vi "PythonFacadeTest.vi"(0 "Data In":T4={"VISA Refnum in"="", "All Code"="Hi"}, 2 "Display State In":T2, 3 "Container State":T3) -> (6 "Data Out":T4={"VISA Refnum in"="", "All Code"="Hi"}, 7 "Display State Out":T2, 8 "Action":T1)   [LabVIEW 2016]
uses:
  <vilib>/_xctls/Action.ctl
  <vilib>/_xctls/XControlSupport.lvlib
  uPythonX.xctl
  <vilib>/_xctls/Container State.ctl
  PythonData.ctl
  PythonState.ctl
panel:
  in  "View":u16(ring)
  in  "SubCode":string
  in  "Save on MP":bool
  in  "REPL":bool
  out "Port":string
  in  "Help":bool
  in  "Python":T5
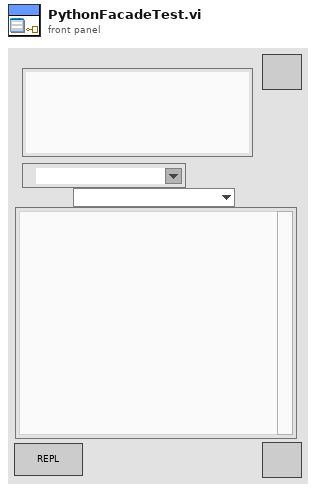
[diagram p1: front panel]
types:
  T1 = typedef "XControlSupport.lvlib/Action.ctl" = cluster{"Data Changed?":bool, "State Changed?":bool, "Action Name":string}
  T2 = typedef "uPythonX.xctl/PythonState.ctl" = cluster{"Numeric":dbl}
  T3 = typedef "XControlSupport.lvlib/Container State.ctl" = cluster{"Indicator?":bool, "Run Mode?":bool, " Refnum":refnum<vi>}
  T4 = typedef "uPythonX.xctl/PythonData.ctl" = cluster{"VISA Refnum in":refnum<visa-resource-name>, "All Code":string}
  T5 = cluster{"VISA in":refnum<visa-resource-name>, "Code":string}
  T6 = cluster{"SubCode":refnum<vi>, "Panel":refnum<vi>}
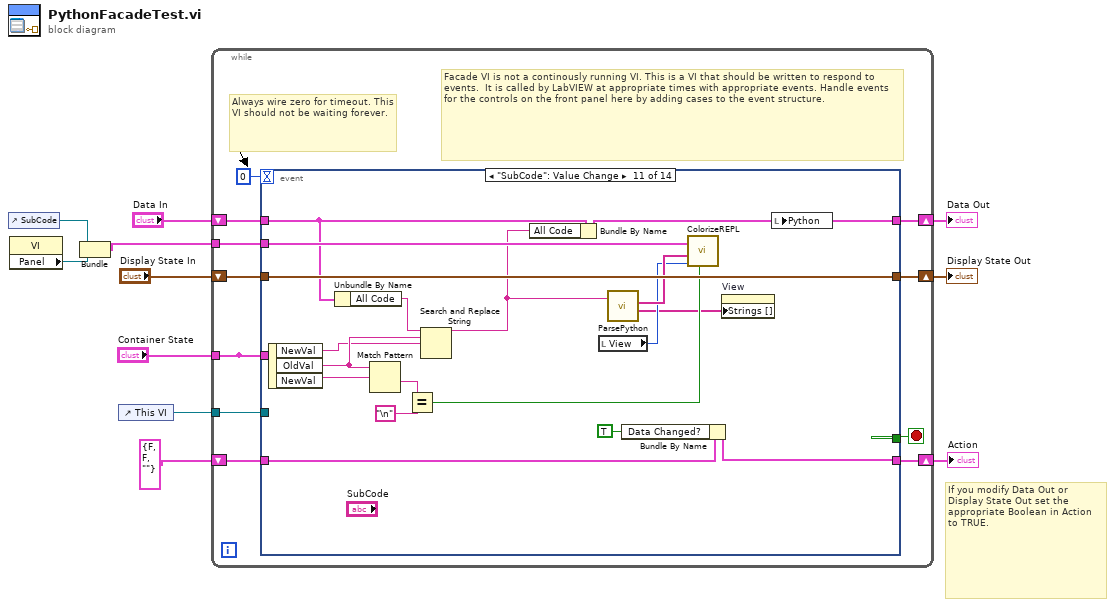
[diagram p0: block diagram]
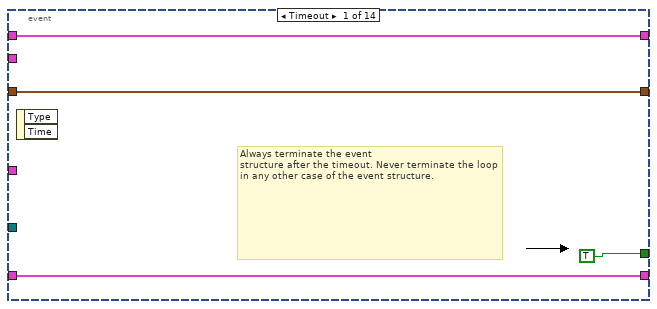
[diagram p2: hidden frame]
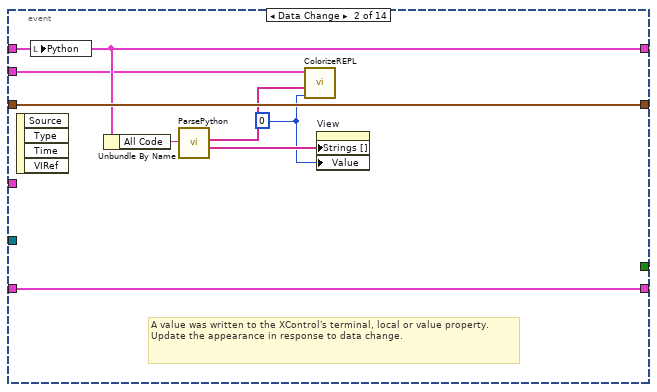
[diagram p3: hidden frame]
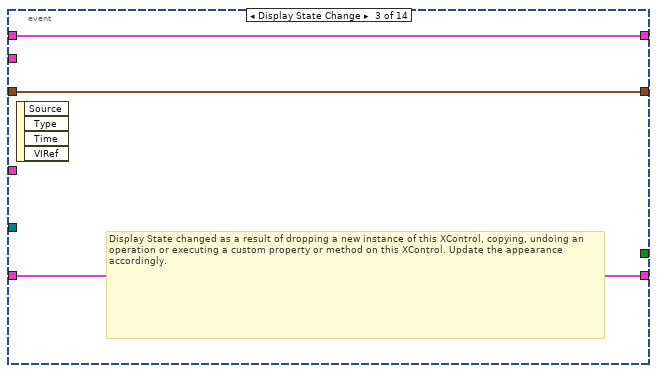
[diagram p4: hidden frame]
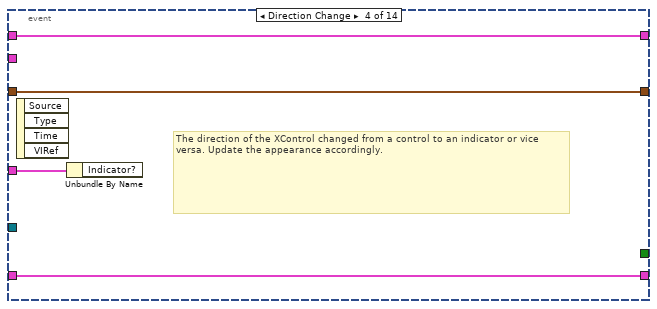
[diagram p5: hidden frame]
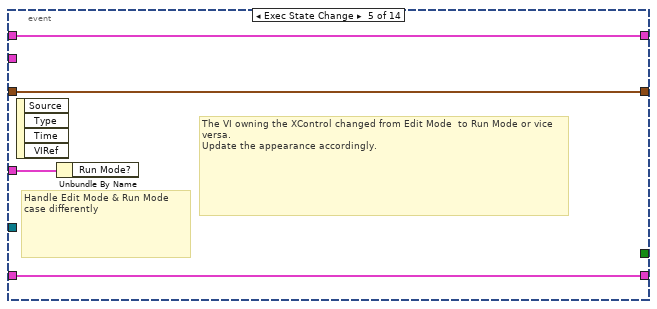
[diagram p6: hidden frame]
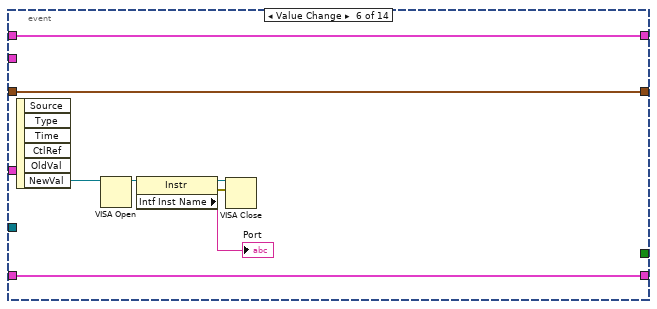
[diagram p7: hidden frame]
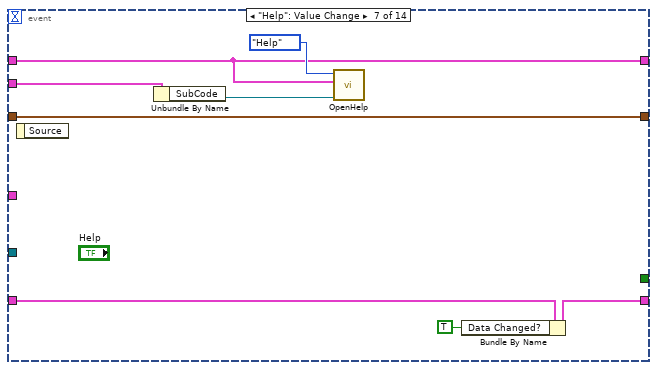
[diagram p8: hidden frame]
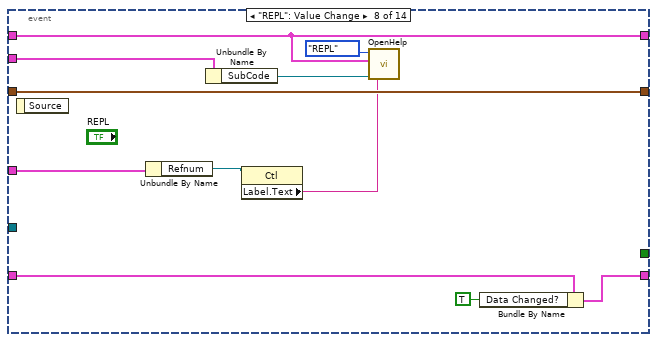
[diagram p9: hidden frame]
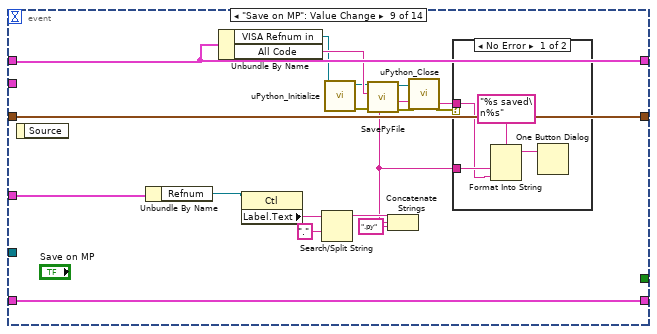
[diagram p10: hidden frame]
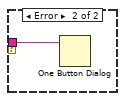
[diagram p11: hidden frame]
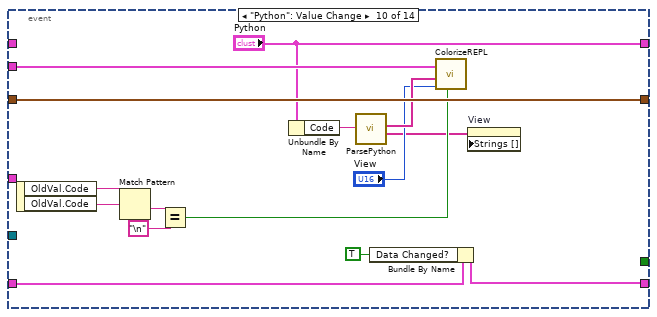
[diagram p12: hidden frame]
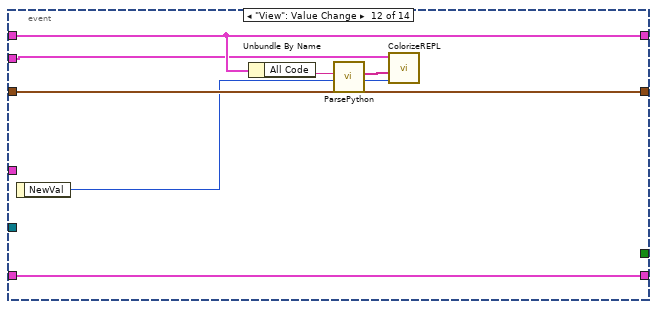
[diagram p13: hidden frame]
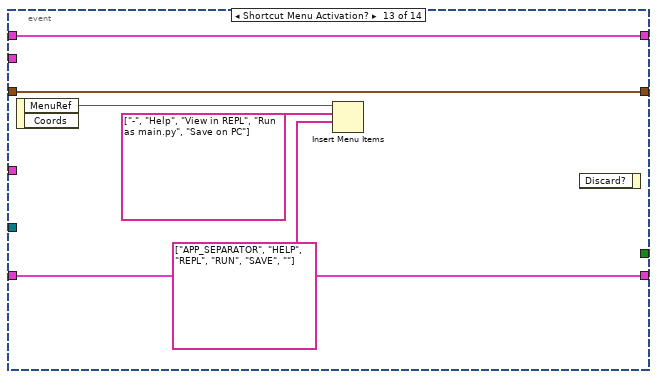
[diagram p14: hidden frame]
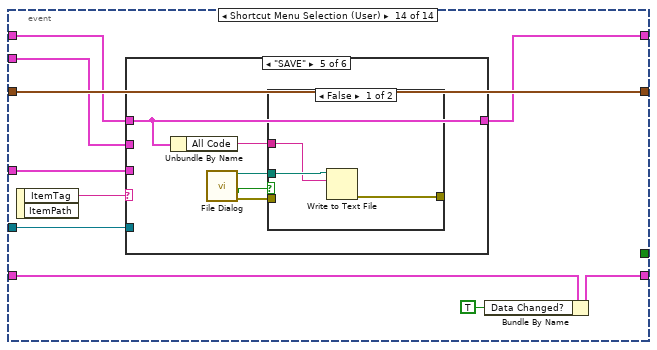
[diagram p15: hidden frame]
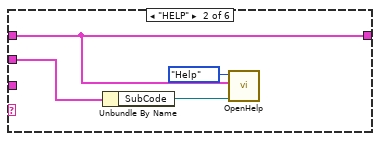
[diagram p17: hidden frame]
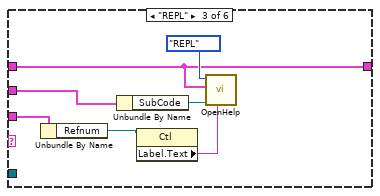
[diagram p18: hidden frame]
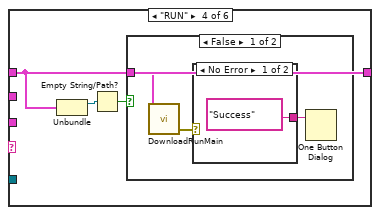
[diagram p19: hidden frame]
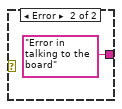
[diagram p20: hidden frame]
diagram:
  # "If you modify Data Out or\nDisplay State Out set the\nappropriate Boolean in Action\nto TRUE."
  n1 = control-ref of="SubCode"() -> (w3:refnum<vi>)
  n2 = property class="VI"() -> ("Panel"=w2:refnum<vi>)  [unwired: 2 in, 2 out]
  n3 = Bundle("SubCode"=w3, "Panel"=w2) -> (w1:T6)  [unwired: 1 in]
  n4 = control-ref of="This VI"() -> (w4:refnum<vi>)
  n5 = while {
    shift-right: [w21] -> w8
    shift-left: "Display State In" -> [w22]
    tunnel: "Container State" -> [w12]
    shift-right: [w17] -> w11
    shift-left: "Data In" -> [w18]
    shift-right: [w15] -> w6
    shift-left: T1 {"Data Changed?"=FALSE, "State Changed?"=FALSE, "Action Name"=""} ("Action") -> [w16]
    tunnel: w4 -> [w14]
    tunnel: w1 -> [w13]
    tunnel: [w12] -> _
    stop <- w20 stop-if-true
    # "Facade VI is not a continously running VI. This is a VI that should be written to respond to events.  It is called by LabVIEW at appropriate times with appropriate events. Handle events for the controls on the front panel here by adding cases to the event structure."
    # "Always wire zero for timeout. This\nVI should not be waiting forever."
    n6 = event shown="[10] \"SubCode\": Value Change" {
      selector: _ -> [_ _ _ _ _ _ _ _ _ _ _ _ _ _]
      dyn-events: _ -> [_ _ _ _ _ _ _ _ _ _ _ _ _ _]
      timeout: 0 -> [_ _ _ _ _ _ _ _ _ _ _ _ _ _]
      tunnel: w22 -> [w24 w34 w37 w40 w44 w53 w61 w72 w90 w110 w128 w135 w141 w151]
      tunnel: [w24 w34 w37 w40 w44 w53 w61 w72 w90 w110 w128 w135 w141 w151] -> w21
      tunnel: [TRUE _ _ _ _ _ _ _ _ _ _ _ _ _] -> w20
      tunnel: w12 -> [_ _ _ w41 w45 _ _ w63 w88 _ _ _ _ w142]
      tunnel: w18 -> [w23 w31 w35 w39 w43 w52 w56 w66 w82 _ w114 w133 w140 w150]
      tunnel: [w23 w31 w35 w39 w43 w52 w56 w66 w82 "Python" w112 w133 w140 w149] -> w17
      tunnel: [w25 w33 w36 w38 w42 w51 w58 w69 w87 w107 w125 w134 w139 w144] -> w15
      tunnel: w16 -> [w25 w33 w36 w38 w42 w51 w59 w70 w87 w109 w127 w134 w139 w145]
      tunnel: w14 -> [_ _ _ _ _ _ _ _ _ _ _ _ _ w147]
      tunnel: w13 -> [_ w29 _ _ _ _ w55 w68 _ w101 w120 w130 _ w143]
      event Timeout {
        # "Always terminate the event\nstructure after the timeout. Never terminate the loop in any other case of the event structure."
        n7 = event-data() -> ()  [unwired: 1 in, 2 out]
      }
      event Data Change {
        w28 = 0
        # "A value was written to the XControl's terminal, local or value property.\nUpdate the appearance in response to data change."
        n8 = event-data() -> ()  [unwired: 1 in, 4 out]
        n9 = local write "Python"(w31) -> ()
        n10 = Unbundle By Name(w31) -> ("All Code"=w30:string)
        n11 = call "ParsePython.vi"("String"=w30) -> ("functions"=w32:string[], "Subs"=w27:string[])  [unwired: 8 in, 1 out]
        n12 = call "ColorizeREPL.vi"("refs"=w29, 2:w27, 3:w28) -> ()  [unwired: 7 in, 1 out]
        n13 = property on="View" class="Ring (strict)"("Strings []"=w32, "Value"=w28) -> ()  [unwired: 2 in, 2 out]
      }
      event Display State Change {
        # "Display State changed as a result of dropping a new instance of this XControl, copying, undoing an operation or executing a custom property or method on this XControl. Update the appearance accordingly."
        n14 = event-data() -> ()  [unwired: 1 in, 4 out]
      }
      event Direction Change {
        # "The direction of the XControl changed from a control to an indicator or vice versa. Update the appearance accordingly."
        n15 = event-data() -> ()  [unwired: 1 in, 4 out]
        n16 = Unbundle By Name(w41) -> ()  [unwired: 1 out]
      }
      event Exec State Change {
        # "The VI owning the XControl changed from Edit Mode  to Run Mode or vice versa.\nUpdate the appearance accordingly."
        # "Handle Edit Mode & Run Mode\ncase differently"
        n17 = event-data() -> ()  [unwired: 1 in, 4 out]
        n18 = Unbundle By Name(w45) -> ()  [unwired: 1 out]
      }
      event "Python.VISA in": Value Change {
        n19 = event-data() -> ("NewVal"=w47:refnum<visa-resource-name>)  [unwired: 1 in, 5 out]
        n20 = VISA Open(VISA resource name=w47) -> (VISA resource name=w48:refnum<visa-resource-name>)  [unwired: 4 in, 1 out]
        n21 = property class="Instr"(reference=w48) -> (reference out=w50:refnum<visa-resource-name>, error out=w49:errorcluster, "Intf Inst Name"=→"Port":string)  [unwired: 1 in]
        n22 = VISA Close(VISA resource name=w50, error in (no error)=w49) -> ()  [unwired: 1 out]
      }
      event "Help": Value Change {
        n23 = event-data() -> ()  [unwired: 1 in, 1 out]
        n24 = Unbundle By Name(w55) -> ("SubCode"=w54:refnum<vi>)
        n25 = call "OpenHelp.vi"("Code Ref"=w54, "Data In"=w56, "Dialog"=enum16{"REPL", "Help"}."Help") -> ()  [unwired: 9 in]
        n26 = Bundle By Name(cluster=w59, "Data Changed?"=TRUE) -> (w58:T1)
      }
      event "REPL": Value Change {
        n27 = event-data() -> ()  [unwired: 1 in, 1 out]
        n28 = Unbundle By Name(w63) -> ("Refnum"=w64:refnum<vi>)
        n29 = Unbundle By Name(w68) -> ("SubCode"=w65:refnum<vi>)
        n30 = property class="Ctl"(reference=w64) -> ("Label.Text"=w62:string)  [unwired: 1 in, 2 out]
        n31 = call "OpenHelp.vi"("Control Name"=w62, "Code Ref"=w65, "Data In"=w66, "Dialog"=enum16{"REPL", "Help"}."REPL") -> ()  [unwired: 8 in]
        n32 = Bundle By Name(cluster=w70, "Data Changed?"=TRUE) -> (w69:T1)
      }
      event "Save on MP": Value Change {
        n33 = event-data() -> ()  [unwired: 1 in, 1 out]
        n34 = Unbundle By Name(w88) -> ("Refnum"=w89:refnum<vi>)
        n35 = Unbundle By Name(w82) -> ("VISA Refnum in"=w78:refnum<visa-resource-name>, "All Code"=w79:string)
        n36 = property class="Ctl"(reference=w89) -> ("Label.Text"=w86:string)  [unwired: 1 in, 2 out]
        n37 = Search/Split String(string=w86, search string/char (-)=".") -> (substring before match=w84:string)  [unwired: 1 in, 2 out]
        n38 = call "uPython_Initialize.vi"("VISA Refnum in"=w78) -> ("error out"=w76:errorcluster, "VISA Refnum out"=w77:refnum<visa-resource-name>)  [unwired: 9 in]
        n39 = Concatenate Strings(w84, ".py" ("string")) -> (w80:string)
        n40 = call "SavePyFile.vi"("Name"=w80, "error in"=w76, "Python Code"=w79, "VISA in"=w77) -> ("error out"=w74:errorcluster, "Reply"=w81:string, "VISA out"=w75:refnum<visa-resource-name>)  [unwired: 5 in]
        n41 = call "uPython_Close.vi"("error in"=w74, "VISA  in"=w75) -> ("error out"=w73:errorcluster)  [unwired: 8 in, 1 out]
        n42 = case shown="No Error" w73 {
          tunnel: w81 -> [w91 w95]
          tunnel: w80 -> [w93 _]
          frame No Error {
            n43 = Format Into String(format string="%s saved\n%s" ("message"), w93, w91) -> (resulting string=w92:string)  [unwired: 2 in, 1 out]
            n44 = One Button Dialog(message=w92) -> ()  [unwired: 1 in, 1 out]
          }
          frame Error {
            n45 = One Button Dialog(message=w95) -> ()  [unwired: 1 in, 1 out]
          }
        }
      }
      event "Python": Value Change {
        n46 = event-data() -> ("OldVal.Code"=w104:string, "OldVal.Code"=w103:string)  [unwired: 1 in]
        n47 = Match Pattern(string=w104, regular expression=w103) -> (after substring=w106:string)  [unwired: 1 in, 3 out]
        n48 = Equal?(x=w106, y="\n") -> (x = y?=w102:bool)
        n49 = Unbundle By Name("Python") -> ("Code"=w98:string)
        n50 = call "ParsePython.vi"("String"=w98) -> ("functions"=w96:string[], "Subs"=w100:string[])  [unwired: 8 in, 1 out]
        n51 = Bundle By Name(cluster=w109, "Data Changed?"=TRUE) -> (w107:T1)
        n52 = call "ColorizeREPL.vi"("refs"=w101, 2:w100, 3:"View", "Add Spaces?"=w102) -> ()  [unwired: 6 in, 1 out]
        n53 = property on="View" class="Ring (strict)"("Strings []"=w96) -> ()  [unwired: 2 in, 2 out]
      }
      event "SubCode": Value Change {
        n54 = event-data() -> ("NewVal"=w116:string, "OldVal"=w117:string, "NewVal"=w122:string)  [unwired: 1 in]
        n55 = Unbundle By Name(w114) -> ("All Code"=w115:string)
        n56 = Match Pattern(string=w117, regular expression=w122) -> (after substring=w124:string)  [unwired: 1 in, 3 out]
        n57 = Equal?(x=w124, y="\n") -> (x = y?=w121:bool)
        n58 = Search and Replace String(input string=w115, search string=w117, replace string=w116) -> (result string=w113:string)  [unwired: 5 in, 3 out]
        n59 = Bundle By Name(cluster=w114, "All Code"=w113) -> (w112:T4)
        n60 = local read "View"() -> (w118:u16)
        n61 = call "ParsePython.vi"("String"=w113) -> ("functions"=w111:string[], "Subs"=w119:string[])  [unwired: 8 in, 1 out]
        n62 = Bundle By Name(cluster=w127, "Data Changed?"=TRUE) -> (w125:T1)
        n63 = call "ColorizeREPL.vi"("refs"=w120, 2:w119, 3:w118, "Add Spaces?"=w121) -> ()  [unwired: 6 in, 1 out]
        n64 = property on="View" class="Ring (strict)"("Strings []"=w111) -> ()  [unwired: 2 in, 2 out]
        n65 = local write "Python"(w112) -> ()
      }
      event "View": Value Change {
        n66 = event-data() -> ("NewVal"=w129:u16)  [unwired: 1 in]
        n67 = Unbundle By Name(w133) -> ("All Code"=w132:string)
        n68 = call "ParsePython.vi"("String"=w132) -> ("Subs"=w131:string[])  [unwired: 8 in, 2 out]
        n69 = call "ColorizeREPL.vi"("refs"=w130, 2:w131, 3:w129) -> ()  [unwired: 7 in, 1 out]
      }
      event "Python.Code": Shortcut Menu Activation? {
        n70 = event-data() -> ("MenuRef"=w136:refnum<k9>)  [unwired: 1 in, 1 out]
        n71 = Insert Menu Items(7:string[] ["APP_SEPARATOR", "HELP", "REPL", "RUN", "SAVE", ""], 8:string[] ["-", "Help", "View in REPL", "Run as main.py", "Save on PC"], 9:w136) -> ()  [unwired: 3 in, 3 out]
        n72 = event-data() -> ()  [unwired: 2 in, 1 out]
      }
      event "Python.Code": Shortcut Menu Selection (User) {
        n73 = event-data() -> ("ItemTag"=w148:string)  [unwired: 1 in, 1 out]
        n74 = case shown="\"SAVE\"" w148 {
          tunnel: w150 -> [w152 w156 w162 w166 w177 w182]
          tunnel: [w152 w156 w162 w166 w177 w181] -> w149
          tunnel: w147 -> [_ _ _ _ _ _]
          tunnel: w143 -> [_ w154 w161 _ _ _]
          tunnel: w142 -> [_ _ w158 _ _ _]
          frame Default {
          }
          frame "HELP" {
            n75 = Unbundle By Name(w154) -> ("SubCode"=w153:refnum<vi>)
            n76 = call "OpenHelp.vi"("Code Ref"=w153, "Data In"=w156, "Dialog"=enum16{"REPL", "Help"}."Help") -> ()  [unwired: 9 in]
          }
          frame "REPL" {
            n77 = Unbundle By Name(w158) -> ("Refnum"=w159:refnum<vi>)
            n78 = Unbundle By Name(w161) -> ("SubCode"=w160:refnum<vi>)
            n79 = property class="Ctl"(reference=w159) -> ("Label.Text"=w157:string)  [unwired: 1 in, 2 out]
            n80 = call "OpenHelp.vi"("Control Name"=w157, "Code Ref"=w160, "Data In"=w162, "Dialog"=enum16{"REPL", "Help"}."REPL") -> ()  [unwired: 8 in]
          }
          frame "RUN" {
            n81 = Unbundle(w166) -> ("VISA Refnum in"=w165:refnum<visa-resource-name>)  [unwired: 1 out]
            n82 = Empty String/Path?(string/path=w165) -> (empty?=w164:bool)
            n83 = case shown="False" w164 {
              tunnel: w166 -> [w169 _]
              frame False {
                n84 = call "DownloadRunMain.vi"("Data In"=w169) -> ("error out"=w167:errorcluster)  [unwired: 8 in, 2 out]
                n85 = case shown="No Error" w167 {
                  tunnel: ["Success" ("message") "Error in talking to the board" ("message")] -> w168
                  frame No Error {
                  }
                  frame Error {
                  }
                }
                n86 = One Button Dialog(message=w168) -> ()  [unwired: 1 in, 1 out]
              }
              frame True {
                n87 = One Button Dialog(message="Select a serial port") -> ()  [unwired: 1 in, 1 out]
              }
            }
          }
          frame "SAVE" {
            n88 = Unbundle By Name(w177) -> ("All Code"=w173:string)
            n89 = call "File Dialog"() -> ("selected path"=w174:path, "cancelled"=w176:bool, "error out"=w175:errorcluster)  [unwired: 12 in, 1 out]
            n90 = case shown="False" w176 {
              tunnel: w175 -> [_ _]
              tunnel: w174 -> [w180 _]
              tunnel: w173 -> [w179 _]
              tunnel: [w178 _] -> _
              frame False {
                n91 = Write to Text File(file (use dialog)=w180, text=w179) -> (error out=w178:errorcluster)  [unwired: 2 in, 2 out]
              }
              frame True {
              }
            }
          }
          frame "REINIT" {
            n92 = invoke on="Python" class="Clust (strict)" method="Reinit To Default"() -> (error out=w183:errorcluster)  [unwired: 3 in, 2 out]
            n93 = case shown="No Error" w183 {
              tunnel: w182 -> [w184 w185]
              tunnel: [w184 w185] -> w181
              frame No Error {
                n94 = local write "Python"(w184) -> ()
              }
              frame Error {
              }
            }
          }
        }
        n95 = Bundle By Name(cluster=w145, "Data Changed?"=TRUE) -> (w144:T1)
      }
    }
  }
  "Display State Out" <- w8
  "Data Out" <- w11
  "Action" <- w6
